vi "SylapExample.vi"() -> ()   [LabVIEW 2020]
panel:
  in  "totalOffset":dbl(slide) caption="Horizontal Pointer Slide" scale=0.0..44961.0
  out "maxPulseLength (ps)":i32
  out "TotalOffset (ps)":dbl
  out "maxPulseLength":i32
  out "Length Pulse (ps)":dbl
  out "TotalOffset (ps) Init":dbl
  in  "pulseLength":u64=10
  out "simLaser freq. (MHz)":dbl
  out "Decimation":dbl
  in  "totalOffset (num) Init":u64
  in  "laserHalfLength":u64=9
  in  "laserMaxCount":u64=10
  in  "VISA resource name":refnum<visa-resource-name>="COM3"
  out "TotalOffset (num)":i32
  # "Initialization parameter"
  # "Loop value"
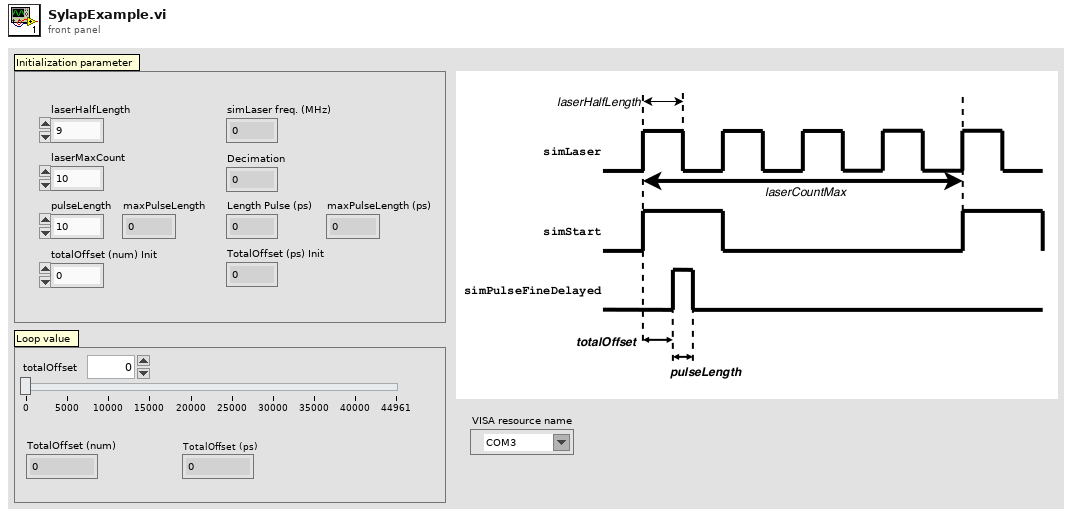
[diagram p1: front panel]
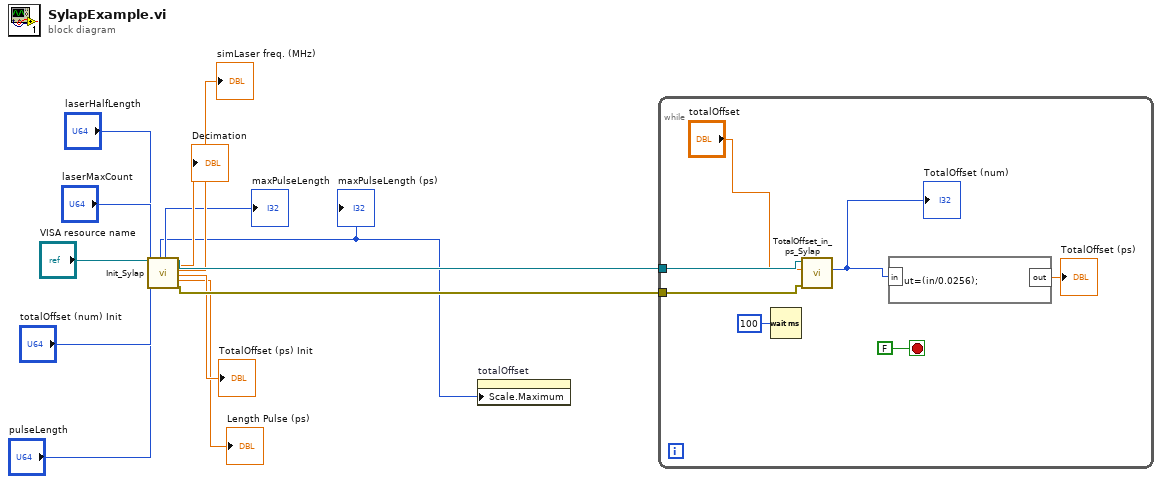
[diagram p0: block diagram]
diagram:
  n1 = call "Init_Sylap.vi"("VISA resource name"="VISA resource name", "LaserMaxCount"="laserMaxCount", "LaserHalfLength"="laserHalfLength", "TotalOffset"="totalOffset (num) Init", "PulseLength"="pulseLength") -> ("maxPulseLength (ps)"=w1:i32, "maxPulseLength"=→"maxPulseLength":i32, "VISA resource name out"=w12:refnum<visa-resource-name>, "Decimation"=→"Decimation":dbl, "simLaser freq. (MHz)"=→"simLaser freq. (MHz)":dbl, "TotalOffset (ps)"=→"TotalOffset (ps) Init":dbl, "Length Pulse (ps)"=→"Length Pulse (ps)":dbl, "error out"=w13:errorcluster)  [unwired: 7 in]
  "maxPulseLength (ps)" <- w1
  n2 = property on="totalOffset" class="Slide (strict)"("Scale.Maximum"=w1) -> ()  [unwired: 2 in, 2 out]
  n3 = while {
    tunnel: w13 -> [w20]
    tunnel: w12 -> [w19]
    stop <- FALSE stop-if-true
    n4 = Wait (ms)(milliseconds to wait=u32 100) -> ()  [unwired: 1 out]
    n5 = call "TotalOffset_in_ps_Sylap.vi"("error in (no error)"=w20, "TotalOffset (ps)"="totalOffset", "VISA resource name"=w19) -> ("TotalOffset (num)"=w16:i32)  [unwired: 6 in, 2 out]
    "TotalOffset (num)" <- w16
    n6 = formula code="out=(in/0.0256);"("in"=w16) -> ("out"=→"TotalOffset (ps)":dbl)
  }
